vi "FpgaLink_Load_Std_Fw.vi"(6 "Timeout in ms (5000)":u32=5000, 8 "error in (no error)":errorcluster, 9 "JTAG Port (D0234)":string="D0234", 10 "New VP (VP)":string, 11 "VP":string) -> (0 "error out":errorcluster, 3 "New VP":string)   [LabVIEW 2011]
doc: "Load standard FPGALink firmware into the FX2's RAM.\n\nLoad the FX2 chip at the \"current\" VID/PID with a precompiled firmware such that it will renumerate as the \"new\" VID/PID. The firmware is loaded into RAM, so the change is not permanent."
uses:
  <vilib>/Utility/importsl/GetValueByPointer/datatype.ctl
  <vilib>/Utility/importsl/GetValueByPointer/GetValueByPointer.xnode
  resource/lvimptsl.dll
  libfpgalink.dll
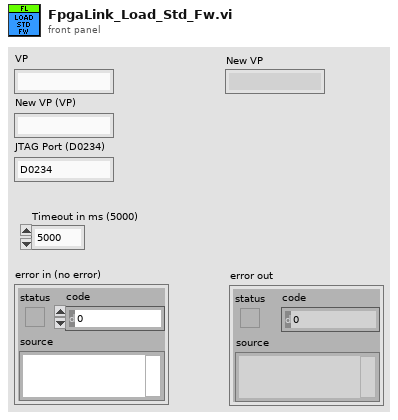
[diagram p1: front panel]
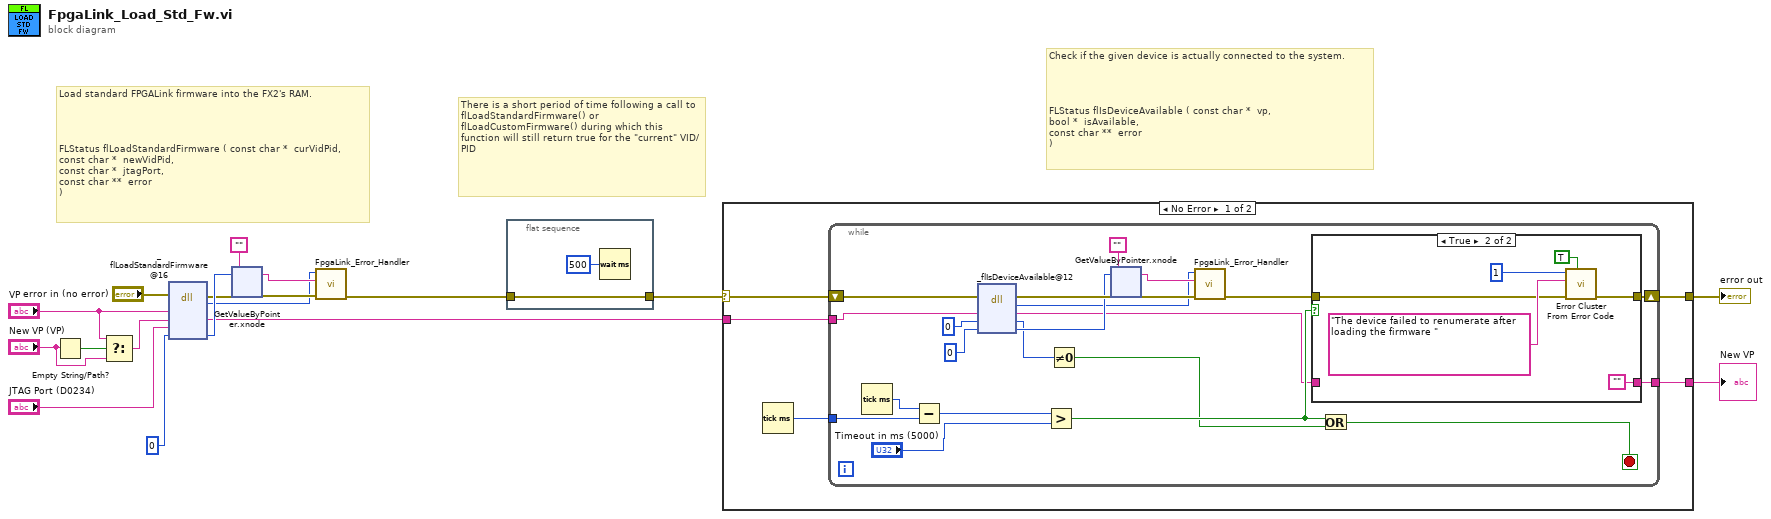
[diagram p0: block diagram]
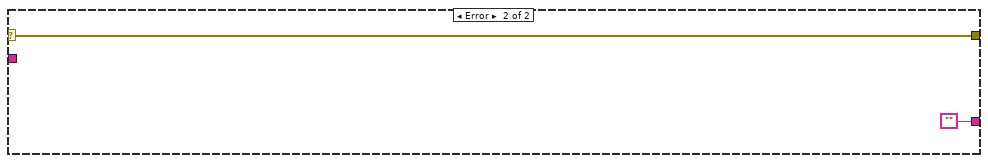
[diagram p3: hidden frame]
diagram:
  # "There is a short period of time following a call to flLoadStandardFirmware() or flLoadCustomFirmware() during which this function will still return true for the \"current\" VID/PID"
  # "Check if the given device is actually connected to the system.\n\n\n\n\nFLStatus flIsDeviceAvailable\t(\tconst char * \tvp,\nbool * \tisAvailable,\nconst char ** \terror \n)"
  # "Load standard FPGALink firmware into the FX2's RAM.\n\n\n\n\nFLStatus flLoadStandardFirmware\t(\tconst char * \tcurVidPid,\nconst char * \tnewVidPid,\nconst char * \tjtagPort,\nconst char ** \terror \n)"
  n1 = Empty String/Path?(string/path="New VP (VP)") -> (empty?=w12:bool)
  n2 = Select(t="VP", s=w12, f="New VP (VP)") -> (s? t:f=w9:string)
  n3 = dll-call lib="libfpgalink.*" fn="_flLoadStandardFirmware@16"(error in="error in (no error)", "curVidPid"="VP", "newVidPid"=w9, "jtagPort"="JTAG Port (D0234)", "error"=i64 0) -> (error out=w15:errorcluster, "FLStatus"=w4:u32, "newVidPid"=w6:string, "error"=w16:i64)  [unwired: 4 in, 1 out]
  n4 = xnode "GetValueByPointer.xnode"("Pointer"=w16, "InputType"="", "ErrorIn"=w15) -> ("Output"=w13:string, "ErrorOut"=w14:errorcluster)  [unwired: 1 in]
  n5 = call <vilib>:"FpgaLink_Error_Handler.vi"("error in (no error)"=w14, "error string"=w13, "error code"=w4) -> ("error out"=w2:errorcluster)  [unwired: 8 in]
  n6 = flat-sequence {
    tunnel: w2 -> [w20]
    tunnel: [w20] -> w1
    frame #0 {
      n7 = Wait (ms)(milliseconds to wait=u32 500) -> ()  [unwired: 1 out]
    }
  }
  n8 = case shown="No Error" w1 {
    selector: w1 -> [w21 w65]
    tunnel: [w23 w65] -> w7
    tunnel: w6 -> [w24 _]
    tunnel: [w22 ""] -> w3
    frame No Error {
      n9 = Tick Count (ms)() -> (millisecond timer value=w25:u32)
      n10 = while {
        shift-right: [w42] -> w23
        shift-left: w21 -> [w47]
        tunnel: w25 -> [w46]
        tunnel: w24 -> [w31]
        tunnel: [w29] -> w22
        stop <- w33 stop-if-true
        n11 = Tick Count (ms)() -> (millisecond timer value=w45:u32)
        n12 = Subtract(x=w45, y=w46) -> (x-y=w44:u32)
        n13 = dll-call lib="libfpgalink.*" fn="_flIsDeviceAvailable@12"(error in=w47, "vp"=w31, "isAvailable"=u8 0, "error_out"=i64 0) -> (error out=w38:errorcluster, "FLStatus"=w34:u32, "vp"=w30:string, "isAvailable"=w27:u8, "error_out"=w35:i64)  [unwired: 2 in, 1 out]
        n14 = Greater?(x=w44, y="Timeout in ms (5000)") -> (0:w32:bool)
        n15 = Not Equal To 0?(x=w27) -> (x != 0?=w26:bool)
        n16 = xnode "GetValueByPointer.xnode"("Pointer"=w35, "InputType"="", "ErrorIn"=w38) -> ("Output"=w40:string, "ErrorOut"=w37:errorcluster)  [unwired: 1 in]
        n17 = call <vilib>:"FpgaLink_Error_Handler.vi"("error in (no error)"=w37, "error string"=w40, "error code"=w34) -> ("error out"=w36:errorcluster)  [unwired: 8 in]
        n18 = case shown="True" w32 {
          tunnel: w36 -> [w57 w59]
          tunnel: [w57 w60] -> w42
          tunnel: w30 -> [w56 _]
          tunnel: [w56 ""] -> w29
          frame False {
          }
          frame True {
            n19 = call <vilib>:"Error Cluster From Error Code.vi"("show call chain? (False)"=TRUE, "error in (no error)"=w59, "error message (\"\")"="The device failed to renumerate after loading the firmware " ("source"), "error code (0)"=1 ("code")) -> ("error out"=w60:errorcluster)  [unwired: 5 in]
          }
        }
        n20 = Or(x=w32, y=w26) -> (x .or. y?=w33:bool)
      }
    }
    frame Error {
    }
  }
  "error out" <- w7
  "New VP" <- w3
